vi "Switch Configuration - Move All Channels.vi"(8 "error in (no error)":errorcluster, 10 "Destiny Listbox Ref In":refnum<vi>, 11 "Origin ListBox Ref In":refnum<vi>) -> (0 "error out":errorcluster, 2 "Destiny ListBox Ref Out":refnum<vi>, 3 "Origin ListBox Ref Out":refnum<vi>, 4 "Destiny Item Names":string[](array[string]), 6 "Origin Item Names":string[](array[string]))   [LabVIEW 2015, in "DMM-SWITCH-ScanList System Explorer.lvlib"]
doc: "Copies current Channel Array from Origin ListBox to Destiny ListBox and deletes Channel Array from Origin ListBox afterwards."
uses:
  DMM-SWITCH-ScanList System Explorer.lvlib
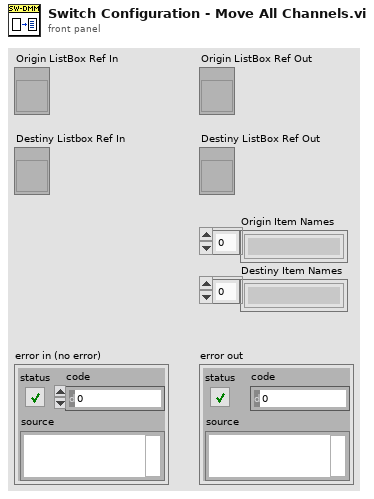
[diagram p1: front panel]
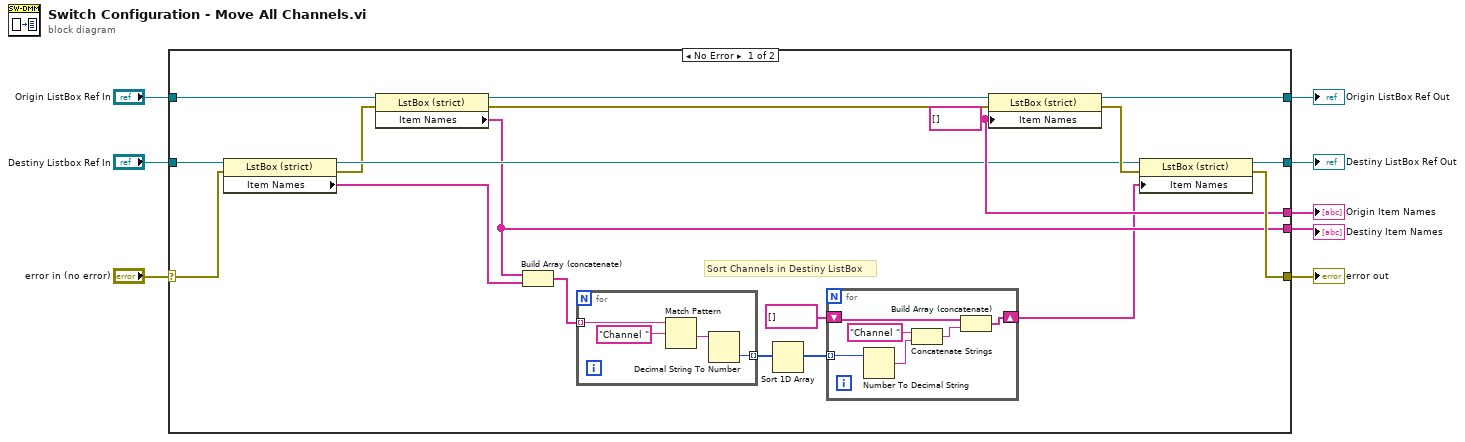
[diagram p0: block diagram]
diagram:
  n1 = case shown="No Error" "error in (no error)" {
    selector: "error in (no error)" -> [w17 w40]
    tunnel: [w27 w40] -> w8
    tunnel: "Origin ListBox Ref In" -> [w22 w39]
    tunnel: [w26 w39] -> w6
    tunnel: [w24 w38] -> w5
    tunnel: "Destiny Listbox Ref In" -> [w19 w38]
    tunnel: [w23 _] -> w2
    tunnel: [w11 _] -> w1
    frame No Error {
      w23 = string[] [] ("Item Names")
      # "Sort Channels in Destiny ListBox"
      n2 = property class="LstBox (strict)"(reference=w19, error in=w17) -> (reference out=w18:refnum<vi>, error out=w16:errorcluster, "Item Names"=w10:string[])
      n3 = property class="LstBox (strict)"(reference=w22, error in=w16) -> (reference out=w21:refnum<vi>, error out=w20:errorcluster, "Item Names"=w11:string[])
      n4 = Build Array (concatenate)(w11, w10) -> (w15:string[])
      n5 = for {
        tunnel: w15 -> [w36] mode=indexing
        tunnel: [w34] -> w12 mode=indexing
        n6 = Match Pattern(string=w36, regular expression="Channel ") -> (after substring=w35:string)  [unwired: 1 in, 3 out]
        n7 = Decimal String To Number(string=w35) -> (number=w34:i32)  [unwired: 2 in, 1 out]
      }
      n8 = Sort 1D Array(array=w12) -> (sorted array=w13:i32[])
      n9 = for {
        tunnel: w13 -> [w33] mode=indexing
        shift-right: [w28] -> w9
        shift-left: string[] [] ("array w/ subset deleted") -> [w32]
        n10 = Number To Decimal String(number=w33) -> (decimal integer string=w29:string)  [unwired: 1 in]
        n11 = Concatenate Strings("Channel " ("string"), w29) -> (w31:string)
        n12 = Build Array (concatenate)(w32, w31) -> (w28:string[])
      }
      n13 = property class="LstBox (strict)"(reference=w21, error in=w20, "Item Names"=w23) -> (reference out=w26:refnum<vi>, error out=w25:errorcluster)
      n14 = property class="LstBox (strict)"(reference=w18, error in=w25, "Item Names"=w9) -> (reference out=w24:refnum<vi>, error out=w27:errorcluster)
    }
    frame Error {
    }
  }
  "error out" <- w8
  "Origin ListBox Ref Out" <- w6
  "Destiny ListBox Ref Out" <- w5
  "Origin Item Names" <- w2
  "Destiny Item Names" <- w1
